vi "ratelimit.vi"(1 "Rate Limit":i16, 2 "In":i16) -> (0 "Out":i16)   [LabVIEW 2010, in "Wall Follower.lvrbt"]
uses:
  Wall Follower.lvrbt
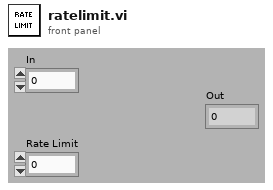
[diagram p1: front panel]
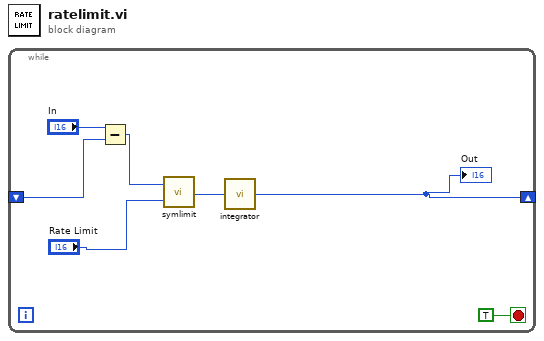
[diagram p0: block diagram]
diagram:
  n1 = while {
    shift-right: [w1] -> _
    shift-left: _ -> [w6]
    stop <- TRUE stop-if-true
    n2 = Subtract(x="In", y=w6) -> (x-y=w4:i16)
    n3 = call "symlimit.vi"("Limit"="Rate Limit", "Input Sig"=w4) -> ("Output Sig"=w2:i16)
    n4 = call "integrator.vi"("In"=w2) -> ("Out"=w1:i16)
    "Out" <- w1
  }
